vi "arduino_test.vi"() -> ()   [LabVIEW 2020]
uses:
  <vilib>/Instr/_visa.llb/VISA Configure Serial Port (Instr).vi
panel:
  in  "arduino COM port":refnum<visa-resource-name>
  out "error out":errorcluster
  in  "Send":bool
  in  "Text To Write":string="1"
  out "read buffer":string
  in  "stop":bool
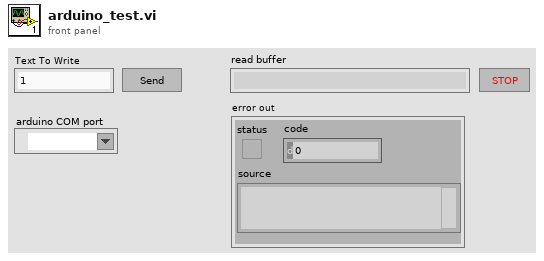
[diagram p1: front panel]
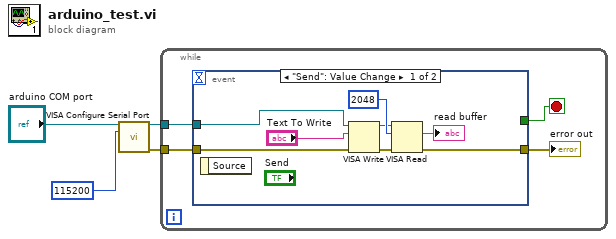
[diagram p0: block diagram]
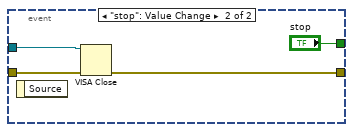
[diagram p2: hidden frame]
diagram:
  n1 = call-poly "VISA Configure Serial Port"("VISA resource name"="arduino COM port", "baud rate (9600)"=115200) -> ("VISA resource name out"=w3:refnum<visa-resource-name>, "error out"=w4:errorcluster)  [unwired: 12 in]
  n2 = while {
    tunnel: w3 -> [w6]
    tunnel: w4 -> [w8]
    stop <- w5 stop-if-true
    n3 = event shown="[0] \"Send\": Value Change" {
      selector: _ -> [_ _]
      dyn-events: _ -> [_ _]
      timeout: _ -> [_ _]
      tunnel: w6 -> [w13 w18]
      tunnel: w8 -> [w16 w20]
      tunnel: [w14 w19] -> w7
      tunnel: [_ "stop"] -> w5
      event "Send": Value Change {
        n4 = event-data() -> ()  [unwired: 1 in, 1 out]
        n5 = VISA Write(VISA resource name=w13, write buffer="Text To Write", error in (no error)=w16) -> (VISA resource name out=w9:refnum<visa-resource-name>, error out=w15:errorcluster)  [unwired: 1 out]
        n6 = VISA Read(VISA resource name=w9, byte count=u32 2048 ("byte count 2"), error in (no error)=w15) -> (read buffer=→"read buffer":string, error out=w14:errorcluster)  [unwired: 2 out]
      }
      event "stop": Value Change {
        n7 = event-data() -> ()  [unwired: 1 in, 1 out]
        n8 = VISA Close(VISA resource name=w18, error in (no error)=w20) -> (error out=w19:errorcluster)
      }
    }
    "error out" <- w7
  }
